vi "GEvt-Generate Remaining States Log.vi"(0 "CSM Global Log Event":refnum<user-event>, 2 "Remaining States":string="<Remaining States>", 6 "Name(\"\" to use uuid)":string, 7 "Enable?":bool, 10 "CSM:LogFilter.lvclass":refnum<class "LogFilter.lvclass">) -> (14 "CSM Global Log Event out":refnum<user-event>, 16 "event data":T1={"Name(\"\" to use uuid)"="", "Current State"="", "Arguments"="", "Source Message"={"‘State"="", "’Arguments"="", "’Error"={"status"=FALSE, "code"=0, "source"=""}}, "Source Module"="", "Complete(T)/Start(F)"=FALSE, "LogType"=enum."State Change"})   [LabVIEW 2020, in "Communicable State Machine.lvlib"]
uses:
  Communicable State Machine.lvlib
  _CSM_GlobalLog_MSG.ctl
  _CSM_Response Source Message.ctl
  _CSM_GlobalLog_MSG_TYPE.ctl
  LogFilter.lvclass
  Filter Check.vi
  Group Check - CSM.vi
  Group Check - LogType.vi
  Group Check - State.vi
  CSM Check - LogType.vi
  CSM Check - State.vi
  CSM Check - StateType.vi
  Group Check - StateType.vi
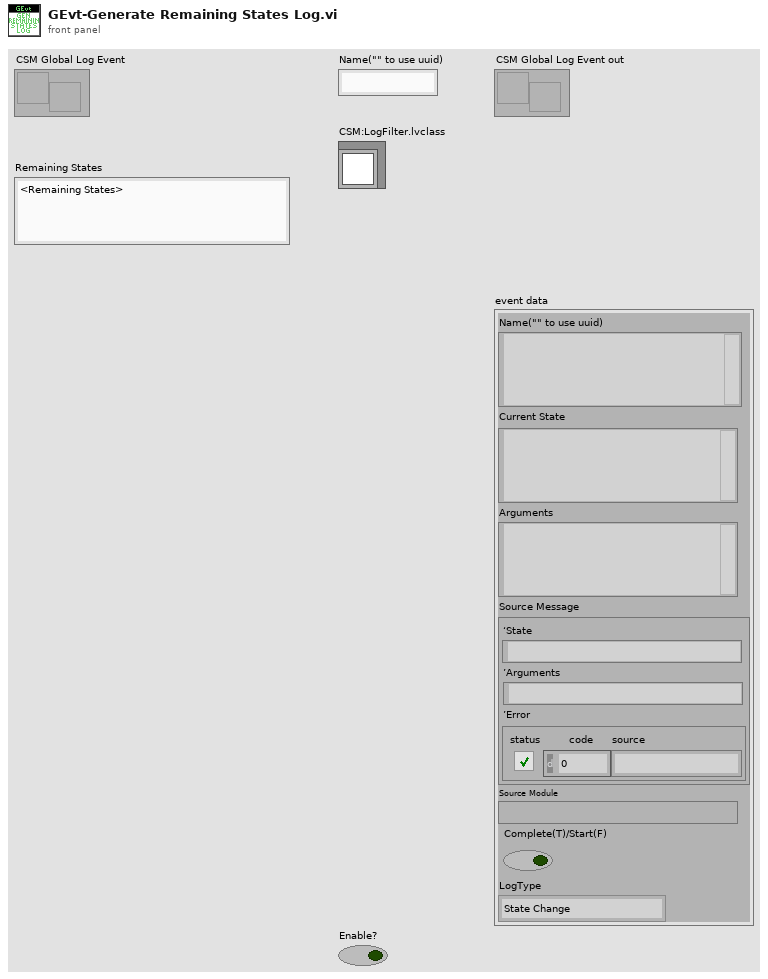
[diagram p1: front panel]
types:
  T1 = typedef "Communicable State Machine.lvlib/_CSM_GlobalLog_MSG.ctl" = cluster{"Name(\"\" to use uuid)":string, "Current State":string, "Arguments":string, "Source Message":T2, "Source Module":string, "Complete(T)/Start(F)":bool, "LogType":T3}
  T2 = typedef "Communicable State Machine.lvlib/_CSM_Response Source Message.ctl" = cluster{"‘State":string, "’Arguments":string, "’Error":errorcluster}
  T3 = typedef "Communicable State Machine.lvlib/_CSM_GlobalLog_MSG_TYPE.ctl" = enum16{"User Log", "State Change", "Status", "Interrupt", "Register", "Unregister", "Error Log", "Module Created", "Module Destroyed"}
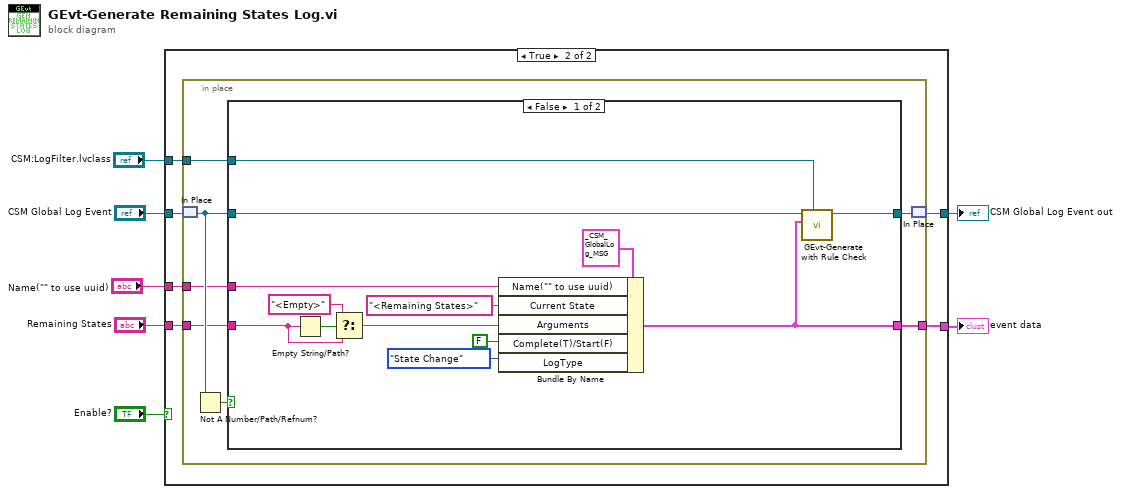
[diagram p0: block diagram]
diagram:
  n1 = case shown="True" "Enable?" {
    tunnel: "CSM Global Log Event" -> [w8 w14]
    tunnel: [w8 w13] -> w6
    tunnel: [_ w12] -> w4
    tunnel: "Name(\"\" to use uuid)" -> [_ w11]
    tunnel: "Remaining States" -> [_ w10]
    tunnel: "CSM:LogFilter.lvclass" -> [_ w9]
    frame False {
    }
    frame True {
      n2 = in-place {
        in-place-border: [w18] -> w12
        in-place-border: w11 -> [w17]
        in-place-border: w10 -> [w16]
        in-place-border: w9 -> [w15]
        n3 = in-place-match #1(w14) -> (w20:refnum<user-event>)
        n4 = Not A Number/Path/Refnum?(number/path/refnum=w20) -> (NaN/Path/Refnum?=w21:bool)
        n5 = case shown="False" w21 {
          tunnel: w20 -> [w34 w35]
          tunnel: [w33 w35] -> w19
          tunnel: [w22 _] -> w18
          tunnel: w17 -> [w25 _]
          tunnel: w16 -> [w24 _]
          tunnel: w15 -> [w23 _]
          frame False {
            n6 = Empty String/Path?(string/path=w24) -> (empty?=w27:bool)
            n7 = Select(t="<Empty>" ("Current State"), s=w27, f=w24) -> (s? t:f=w26:string)
            n8 = Bundle By Name(cluster=T1 {"Name(\"\" to use uuid)"="", "Current State"="", "Arguments"="", "Source Message"={"‘State"="", "’Arguments"="", "’Error"={"status"=FALSE, "code"=0, "source"=""}}, "Source Module"="", "Complete(T)/Start(F)"=FALSE, "LogType"=enum."State Change"} ("event data"), "Name(\"\" to use uuid)"=w25, "Current State"="<Remaining States>", "Arguments"=w26, "Complete(T)/Start(F)"=FALSE, "LogType"=_CSM_GlobalLog_MSG_TYPE."State Change" ("Type")) -> (w22:T1)
            n9 = call "GEvt-Generate with Rule Check.vi"("LogFilter in"=w23, "event data"=w22, "CSM Global Log Event in"=w34) -> ("CSM Global Log Event out"=w33:refnum<user-event>)  [unwired: 8 in]
          }
          frame True {
          }
        }
        n10 = in-place-match #1(w19) -> (w13:refnum<user-event>)
      }
    }
  }
  "CSM Global Log Event out" <- w6
  "event data" <- w4
